vi "ErrorScreen.vi"(8 "error in":errorcluster) -> (0 "error out":errorcluster)   [LabVIEW 2011]
uses:
  SubVIs/Controls/TransparencyEffectOperations.ctl
panel:
  in  "INIT":bool
  in  "STOP":bool
  # "Lost Connection to the Chassis or Module! Please connect your Device and Start Again!"
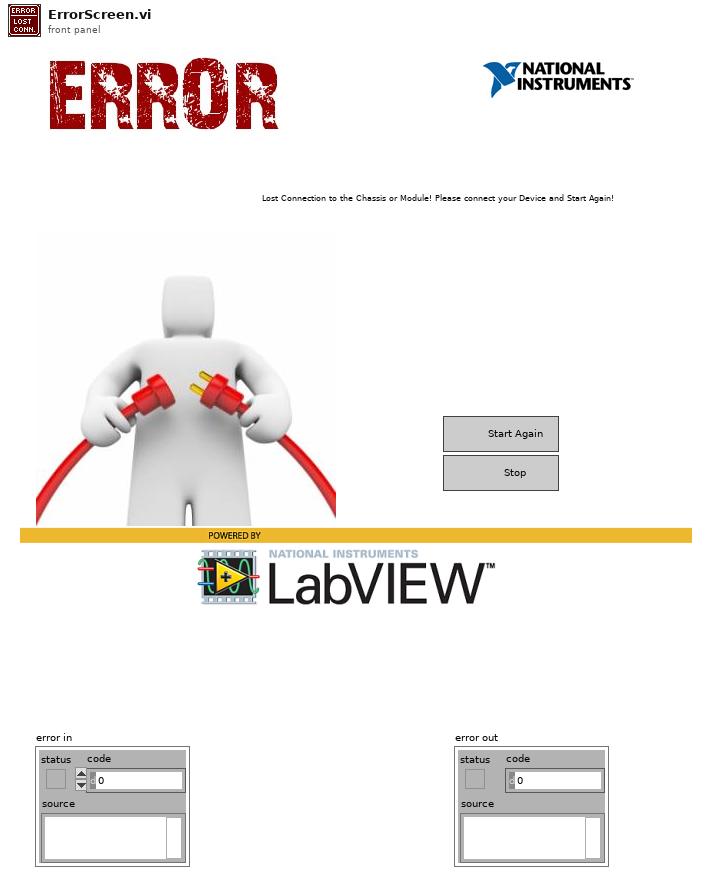
[diagram p1: front panel]
types:
  T1 = typedef "TransparencyEffectOperations.ctl" = enum16{"Show", "Hide 80%", "Hide All"}
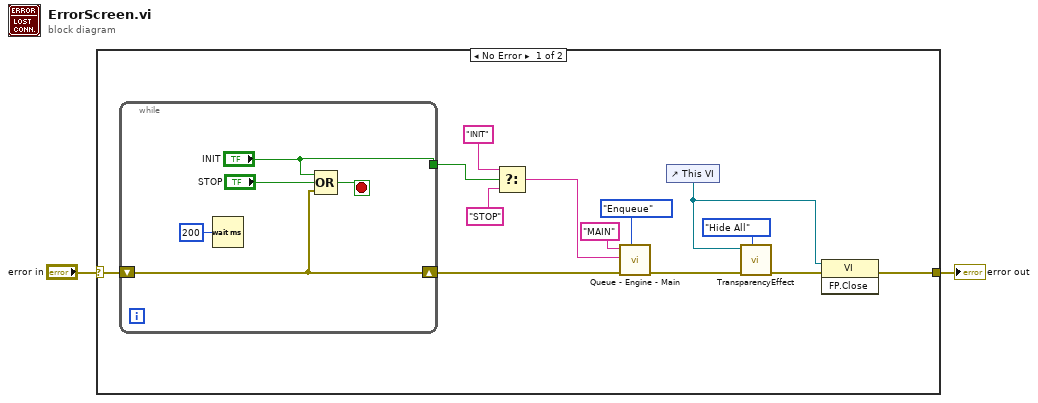
[diagram p0: block diagram]
diagram:
  n1 = case shown="No Error" "error in" {
    selector: "error in" -> [w15 w21]
    tunnel: [w4 w21] -> w2
    frame No Error {
      n2 = while {
        shift-right: [w17] -> w12
        shift-left: w15 -> [w17]
        tunnel: ["INIT"] -> w9
        stop <- w16 stop-if-true
        n3 = Wait (ms)(milliseconds to wait=u32 200) -> ()  [unwired: 1 out]
        n4 = Compound Arithmetic op=OR("INIT", "STOP", w17) -> (w16:bool)
      }
      n5 = Select(t="INIT" ("Queue Name In"), s=w9, f="STOP" ("Queue Name In")) -> (s? t:f=w3:string)
      n6 = call "Queue - Engine - Main.vi"("Operation"=enum16{"Enqueue", "Dequeue", "Flush", "Release"}."Enqueue", "error in"=w12, "Queue Data In"=w3, "Queue Name In"="MAIN") -> ("error out"=w7:errorcluster)  [unwired: 5 in, 2 out]
      n7 = control-ref of="This VI"() -> (w6:refnum<vi>)
      n8 = call "TransparencyEffect.vi"("Operation"=TransparencyEffectOperations."Hide All", "error in"=w7, "VI Ref in"=w6) -> ("error out"=w5:errorcluster)  [unwired: 8 in]
      n9 = invoke class="VI" method="FP.Close"(reference=w6, error in=w5) -> (error out=w4:errorcluster)  [unwired: 1 in, 2 out]
    }
    frame Error {
    }
  }
  "error out" <- w2
